vi "QR Code Reader.vi"() -> ()   [LabVIEW 2017]
uses:
  <vilib>/userdefined/High Color/IMAQdx.ctl
  <vilib>/vision/driver/NI_Vision_Acquisition_Software.lvlib
  <vilib>/vision/NI_Vision_Development_Module.lvlib
panel:
  out "error out 2":errorcluster
  out "Data":string
  out "Image":T1(plugin-control)
  out "Found?":bool
  out "error out":errorcluster
  in  "Session In":T2
  in  "stop":bool
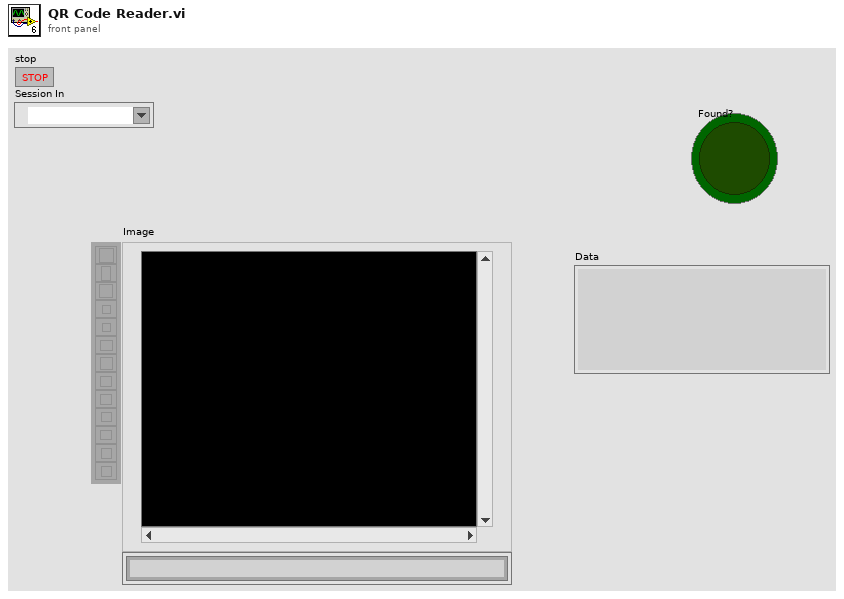
[diagram p1: front panel]
types:
  T1 = typedef "IMAQ Image.ctl" = refnum<image>
  T2 = typedef "IMAQdx.ctl" = refnum<k21>
  T3 = typedef "Image Type" = u32
  T4 = typedef "QR Code Report.ctl" = cluster{"Found?":bool, "Data":string, "Bounding Box":cluster{"x":sgl, "y":sgl}[], "Errors Corrected":u32, "Dimensions (Rows/Cols)":u32, "Version":u32, "QR Model":T5, "Stream Mode":T6, "Barcode Polarity":T7, "Mirrored?":bool, "Append Stream Position":u32, "Size of Append Stream":u32, "First EAN-128 ID":i32, "First Alternate Language ID":i32, "Append Stream ID":u32, "Minimum Edge Strength":u32, "Demodulation Mode":T8, "Cell Sample Size":T9, "Cell Filter Mode":T10}
  T5 = typedef "QR Code Model Type.ctl" = i32
  T6 = typedef "QR Code Stream Mode Type.ctl" = i32
  T7 = typedef "Data Matrix Polarity.ctl" = i32
  T8 = typedef "Demodulation Mode.ctl" = i32
  T9 = typedef "Cell Sample Size.ctl" = i32
  T10 = typedef "Cell Filter Mode.ctl" = i32
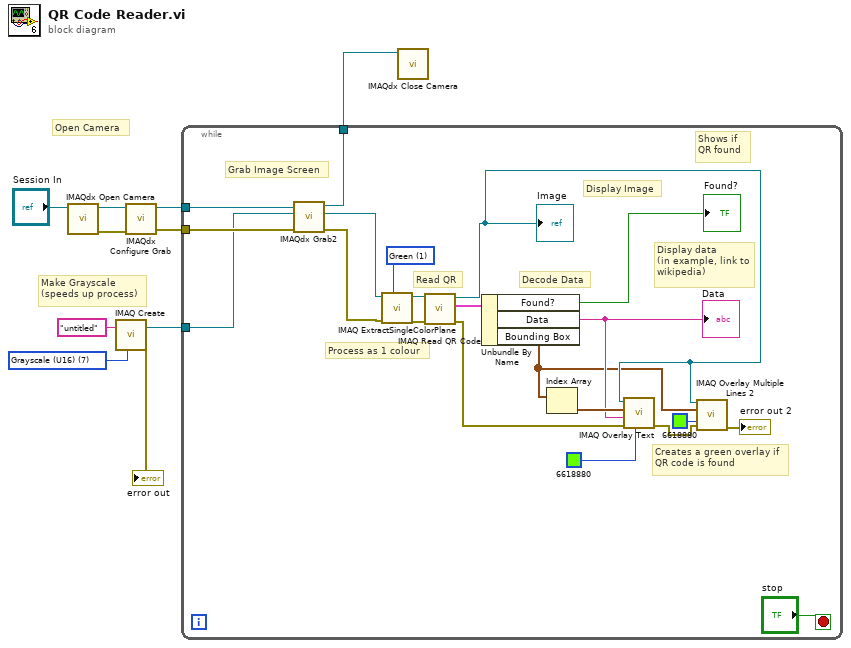
[diagram p0: block diagram]
diagram:
  w3 = T3 7 items=["Grayscale (U8)", "Grayscale (I16)", "Grayscale (SGL)", "Complex (CSG)", "RGB (U32)", "HSL (U32)", "RGB (U64)", "Grayscale (U16)"] ("Image Type")
  # "Make Grayscale\n(speeds up process)"
  # "Open Camera"
  n1 = call <vilib>:"IMAQdx Open Camera.vi"("Session In"="Session In") -> ("error out"=w8:errorcluster, "Session Out"=w9:T2)  [unwired: 9 in]
  n2 = call "IMAQ Create"("Image Name"="untitled", "Image Type"=w3) -> ("New Image"=w2:T1, "error out"=→"error out":errorcluster)  [unwired: 3 in]
  n3 = call <vilib>:"IMAQdx Configure Grab.vi"("error in"=w8, "Session In"=w9) -> ("error out"=w5:errorcluster, "Session Out"=w7:T2)  [unwired: 8 in]
  n4 = while {
    tunnel: w7 -> [w30]
    tunnel: [w29] -> w6
    tunnel: w5 -> [w28]
    tunnel: w2 -> [w27]
    stop <- "stop" stop-if-true
    w22 = 1 items=["Red", "Green", "Blue", "Hue", "Saturation", "Luminance", "Value", "Intensity"] ("Color Plane")
    # "Creates a green overlay if\nQR code is found"
    # "Shows if\nQR found"
    # "Display data\n(in example, link to wikipedia)"
    # "Decode Data"
    # "Display Image"
    # "Read QR"
    # "Process as 1 colour"
    # "Grab Image Screen"
    n5 = call <vilib>:"IMAQdx Grab2.vi"("error in"=w28, "Image In"=w27, "Session In"=w30) -> ("error out"=w23:errorcluster, "Image Out"=w24:T1, "Session Out"=w29:T2)  [unwired: 5 in, 1 out]
    n6 = call "IMAQ ExtractSingleColorPlane"("Color Plane"=w22, "error in (no error)"=w23, "Image Src"=w24) -> ("error out"=w25:errorcluster, "Image Dst Out"=w26:T1)  [unwired: 7 in]
    n7 = call "IMAQ Read QR Code"("error in (no error)"=w25, "Image"=w26) -> ("error out"=w11:errorcluster, "QR Code Report"=w21:T4, "Image (duplicate)"=w16:T1)  [unwired: 6 in, 1 out]
    "Image" <- w16
    n8 = Unbundle By Name(w21) -> ("Found?"=→"Found?":bool, "Data"=w18:string, "Bounding Box"=w15:cluster{"x":sgl, "y":sgl}[])
    "Data" <- w18
    n9 = Index Array(array=w15) -> (element=w19:cluster{"x":sgl, "y":sgl})  [unwired: 1 in]
    n10 = call "IMAQ Overlay Text"("Text Color (black)"=u32 6618880, "error in (no error)"=w11, "String"=w18, "Origin"=w19, "Image"=w16) -> ("error out"=w13:errorcluster)  [unwired: 5 in, 1 out]
    n11 = call "IMAQ Overlay Multiple Lines 2"("Image"=w16, "Line End Points"=w15, "Color"=u32 6618880, "error in (no error)"=w13) -> ("error out"=→"error out 2":errorcluster)  [unwired: 10 in, 1 out]
  }
  n12 = call <vilib>:"IMAQdx Close Camera.vi"("Session In"=w6) -> ()  [unwired: 10 in, 1 out]
